vi "NISE.Commit NVMEM (Core).vi"(7 "nvmem type":T1, 8 "error in (no error)":errorcluster, 10 "resources":string, 11 "SLSC Interface in":refnum<class "SLSC Interface.lvclass">) -> (0 "error out":errorcluster, 3 "SLSC Interface out":refnum<class "SLSC Interface.lvclass">)   [LabVIEW 2016, in "SLSC Interface.lvclass"]
uses:
  SLSC Interface.lvclass
  NISE.nvmem type.ctl
  SLSC Interface.lvclass/SLSC Interface.ctl
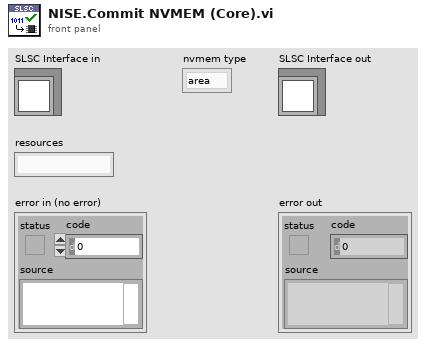
[diagram p1: front panel]
types:
  T1 = typedef "SLSC Interface.lvclass/NISE.nvmem type.ctl" = enum16{"area", "device", "session"}
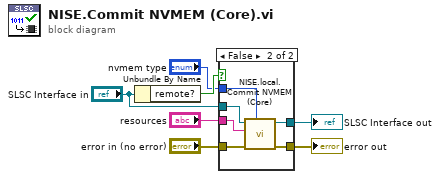
[diagram p0: block diagram]
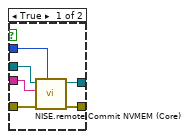
[diagram p2: hidden frame]
diagram:
  n1 = Unbundle By Name("SLSC Interface in") -> ("remote?"=w7:bool)
  n2 = case shown="False" w7 {
    tunnel: [w13 w19] -> w6
    tunnel: [w12 w18] -> w5
    tunnel: "nvmem type" -> [w11 w17]
    tunnel: "error in (no error)" -> [w10 w16]
    tunnel: "resources" -> [w9 w15]
    tunnel: "SLSC Interface in" -> [w8 w14]
    frame True {
      n3 = call "NISE.remote.Commit NVMEM (Core).vi"("nvmem type"=w11, "error in (no error)"=w10, "resources"=w9, "SLSC Remote in"=w8) -> ("error out"=w13:errorcluster, "SLSC Remote out"=w12:refnum<class "SLSC Interface.lvclass">)  [unwired: 6 in]
    }
    frame False {
      n4 = call "NISE.local.Commit NVMEM (Core).vi"("nvmem type"=w17, "error in (no error)"=w16, "resources"=w15, "SLSC Local in"=w14) -> ("error out"=w19:errorcluster, "SLSC Local out"=w18:refnum<class "SLSC Interface.lvclass">)  [unwired: 6 in]
    }
  }
  "error out" <- w6
  "SLSC Interface out" <- w5
